vi "AutoJoystickLogic.vi"() -> (2 "Speeds":dbl[](array[numeric]), 3 "Angles":dbl[](array[numeric]))   [LabVIEW 2017]
uses:
  AutoGlobals.vi
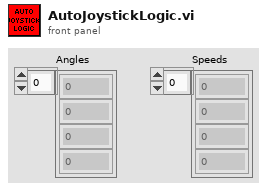
[diagram p1: front panel]
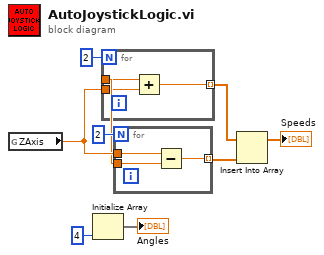
[diagram p0: block diagram]
diagram:
  n1 = global read "AutoGlobals.vi" "ZAxis"() -> (w2:dbl)
  n2 = Initialize Array(4 ("dimension size")) -> (→"Angles":void[])  [unwired: 1 in]
  n3 = for {
    N: 2 -> [_]
    tunnel: [w11] -> w1
    tunnel: w2 -> [w12]
    tunnel: [w10] -> w4 mode=indexing
    n4 = Add(x=w11, y=w12) -> (x+y=w10:dbl)
  }
  n5 = for {
    N: 2 -> [_]
    tunnel: w1 -> [w13]
    tunnel: w2 -> [w14]
    tunnel: [w15] -> w5 mode=indexing
    n6 = Subtract(x=w14, y=w13) -> (x-y=w15:dbl)
  }
  n7 = Insert Into Array(array=w4, new element=w5) -> (→"Speeds":dbl[])  [unwired: 1 in]
